vi "GetDisplayName2.vi"(0 "XRef":T3, 1 "State In":T2) -> (14 "Name":T1)   [LabVIEW 2012, in "OpenG Delete Elements from Array.xnode"]
doc: "This ability VI is used to supply LabVIEW with the name of your XNode. This is used as the default value for the label, it is used to mark entries in the error list and the difference list.\n\nDefault behavior: None.\n\nThis ability does not provide UI and OS messages are not handled."
uses:
  OpenG Delete Elements from Array.xnode
  <vilib>/XNodeSupport/XNodeXNodeRef.ctl
  State.ctl
  <vilib>/XNodeSupport/XNodeString.ctl
  <vilib>/XNodeSupport/NI_XNodeSupport.lvlib
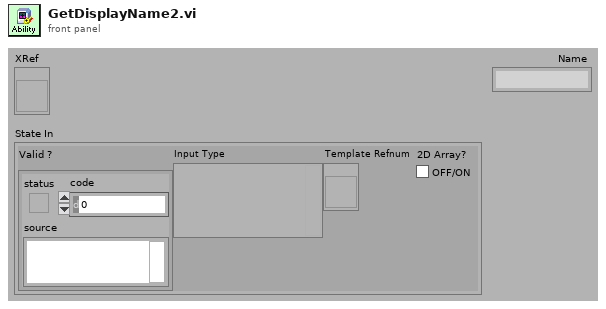
[diagram p1: front panel]
types:
  T1 = typedef "NI_XNodeSupport.lvlib/XNodeString.ctl" = string
  T2 = typedef "OpenG Delete Elements from Array.xnode/State.ctl" = cluster{"Valid ?":errorcluster, "Input Type":variant, "Template Refnum":refnum<vi>, "2D Array?":bool}
  T3 = typedef "NI_XNodeSupport.lvlib/XNodeXNodeRef.ctl" = refnum<vi>
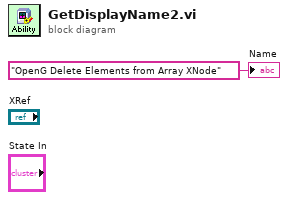
[diagram p0: block diagram]
diagram:
  "Name" <- T1 "OpenG Delete Elements from Array XNode" ("Name")
